vi "Plate Tank 3.vi"() -> ()   [LabVIEW 2019]
uses:
  <vilib>/NI/Current Value Table/Type Defs/Single Tag.ctl
  <vilib>/NI/Current Value Table/Type Defs/Data Types.ctl
  <vilib>/Utility/sysdir.llb/System Directory Type.ctl
  <vilib>/NI/STM/TCP/Read Meta Data (TCP Ref).vi
  <vilib>/NI/STM/TCP/Get Connection Reference (TCP).vi
  <vilib>/NI/AMC/Read Termination Message.vi
  <vilib>/NI/AMC/Create Single Message.vi
  <vilib>/NI/AMC/Update Message Routing Info.vi
  <vilib>/NI/STM/TCP/Read Meta Data (TCP Clst).vi
  <vilib>/NI/AMC/Send Message.vi
  <vilib>/NI/AMC/Globals.vi
  <userlib>/_OpenG.lib/comparison/comparison.llb/I32 Changed__ogtk.vi
  <vilib>/NI/STM/TCP/Write Message (TCP).vi
  <vilib>/NI/AMC/AMC.lvlib
  <vilib>/NI/STM/NI STM.lvlib
  <vilib>/NI/Current Value Table/Current Value Table.lvlib
panel:
  in  "EZ Recipe Button":bool
  out "Loaded Recipe":string
  in  "Load A Recipe":bool
  in  "Save This Recipe":bool
  out "Right Time":dbl format="%.1f"
  out "Left Time":dbl format="%.1f"
  out "Total Amp*min R":dbl format="%.1f"
  out "Total Amp*min L":dbl format="%.1f"
  in  "Rectifer Settings":i32(listbox)
  in  "MO":string
  in  "BasT1_P Last Hr":bool
  in  "BasT1_Level Last Hr":bool
  out "Boolean 5":bool
  out "SumpBottom":bool
  out "Process 1 Supply":bool
  out "Sump Return":bool
  out "Boolean 2":bool
  out "SG":dbl format="%.3g"
  out "Return to sump 4":bool
  in  "Rectifer Data":enum32{"Standard", "Eng"}(tab)
  out "Current Step":i32
  out "Left Anode Actual Current":dbl(knob) scale=0.0..150.0
  out "Right Anode Actual Current":dbl(knob) scale=0.0..150.0
  out "Left Anode Amp-min":dbl(slide) scale=0.0..800.0
  out "Right Anode Amp-min":dbl(slide) scale=0.0..233.60000610351562
  out "Output Voltage":cluster{dbl, dbl}(graph)
  in  "Tab Control 2":enum32{"Standard", "ENG"}(tab)
  out "Supply Flow":dbl(knob) scale=0.0..65.0
  out "Plating Cell Liquid Level":dbl(slide) scale=0.0..75.0
  out "Cell Temperature":dbl(slide) scale=0.0..60.0
  in  "Cell T Last Hr":bool
  out "Suck Pump":bool
  out "Suck Pump Flow":dbl format="%#_4g"
  out "SuckPipe":bool
  out "SuckPipe 3":bool
  out "Drain Tee Top":bool
  out "Return to sump 2":bool
  out "Return to sump 3":bool
  out "Flow Controller":dbl(knob) scale=0.0..100.0
  in  "Tab Control":enum32{"Main Pump", "Suck Pump"}(tab)
  out "Amps":dbl format="%#.2g"
  out "Volts":dbl format="%#.1f"
  out "VFD T":dbl format="%#.2g"
  out "RPM":dbl format="%#.0f"
  out "Fault Code":dbl format="%#.2g"
  out "Freq":dbl format="%#.2g"
  out "SP1 Amps":dbl caption="Amps" format="%#.2g"
  out "SP1 Volts":dbl caption="Volts" format="%#.1g"
  out "SP1 RPM":dbl caption="RPM" format="%#.2g"
  out "SP1 VFD T":dbl caption="VFD T" format="%#.2g"
  out "SP1 Fault Code":dbl caption="Fault Code" format="%#.2g"
  out "SP1 Freq":dbl caption="Freq" format="%#.2g"
  out "Flow 1":dbl format="%#_4g"
  out "Flow 2":dbl format="%#_4g"
  out "Flow 3":dbl format="%#_4g"
  out "Flow 4":dbl format="%#_4g"
  out "Return to sump":bool
  out "E Stop":bool
  out "Run Enabled?":bool
  in  "Full Drain Plating Cell":bool
  out "Rack Motion":bool
  out "Right Eductor Motion":bool
  out "Left Eductor Motion":bool
  out "Right Output On":bool
  in  "Enable Rack Motion":bool
  in  "Rack RPM":dbl(knob) scale=0.0..15.0
  out "Left Output On":bool
  in  "Start Cycle":bool
  in  "Cancel Cycle":bool
  out "SuckPipe 2":bool
  out "Main Pump":bool
  in  "Enable Eductor Motion":bool
  in  "Eductor RPM":dbl(knob) scale=0.0..15.0
  in  "Supply Pressure (kPa)":dbl(knob)=50.0 min=50.0 max=200.0 step=5.0 scale=50.0..200.0
  in  "Total Inflow (L/min)":dbl(knob)=40.0 min=25.0 max=50.0 step=0.5 scale=25.0..50.0
  in  "Suck Pump fraction of inflow":dbl(knob)=5.0 min=5.0 max=90.0 step=1.0 scale=0.0..90.0
  out "Sump Level":dbl(slide) scale=0.0..1000.0
  out "Supply Pressure":dbl(knob) scale=0.0..200.0
  in  "Enable Suck Pump":bool
  in  "Enable Plating Cell":bool
  in  "Machine":bool
  in  "Basement 4":bool
  in  "Dryer":bool
  in  "Rinse 4":bool
  in  "Rinse 3":bool
  in  "Rinse 2":bool
  in  "Basement 3":bool
  in  "Basement 2":bool
  in  "Basement 1":bool
  in  "Plater 6":bool
  in  "Plater 5":bool
  in  "Plater 4":bool
  in  "Plater 3":bool
  in  "Plater 2":bool
  in  "Plater 1":bool
  in  "Predip":bool
  in  "Rinse 1":bool
  in  "Cleaner":bool
  in  "Etch":bool
  out "status":string
  out "Boolean 4":bool
  # "Module Selection"
  # "Rectifier Settings"
  # "Recipe"
  # "Fluid Flow Control"
  # "Rectifier Control"
  # "Rectifier Output"
  # "Motion starts when rectifiers cycle"
  # "Note: RPM settings shared with tank 4"
  # "kPa"
  # "@"
  # "Output"
  # "cm"
  # "°C"
  # "L/min"
  # "cm"
  # "L/min"
  # "L/min"
  # "L/min"
  # "L/min"
  # "L/min"
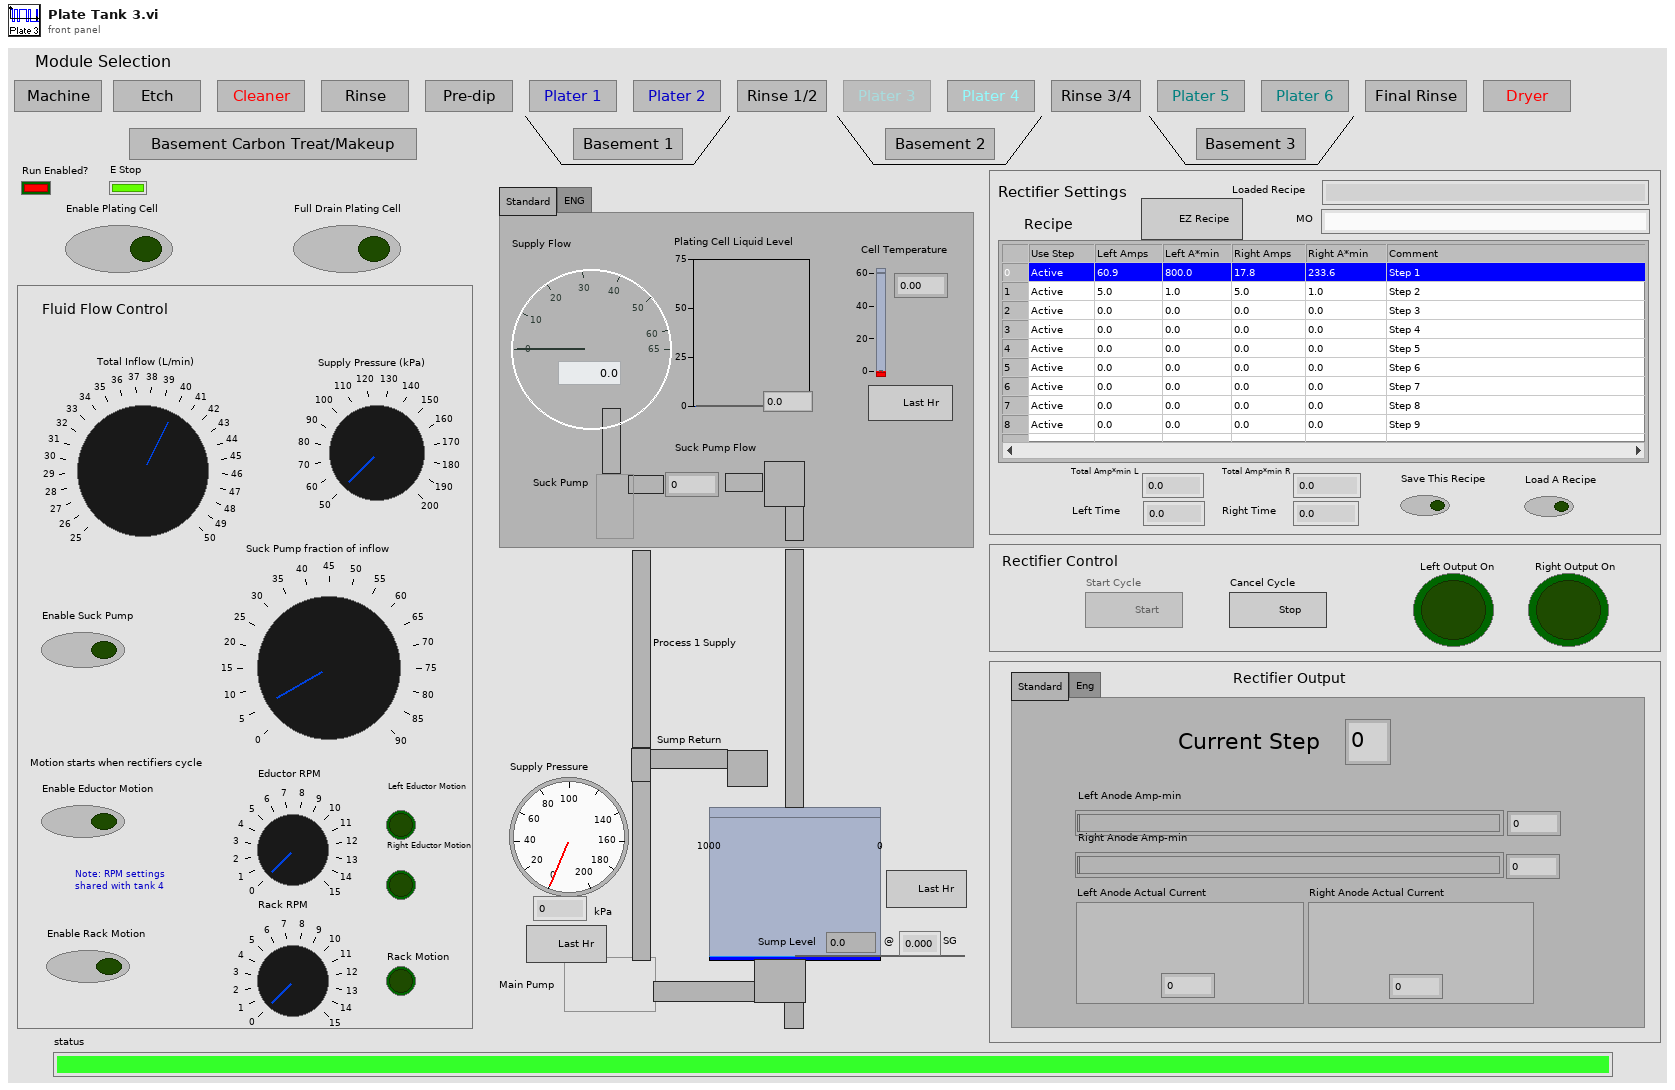
[diagram p1: front panel]
types:
  T1 = typedef "Current Value Table.lvlib/Single Tag.ctl" = cluster{"Data Type":T2, "Name":string, "Value":string, "Description":string}
  T2 = typedef "Current Value Table.lvlib/Data Types.ctl" = enum16{"Double", "Single", "I64", "I32", "I16", "I8", "U64", "U32", "U16", "U8", "String", "Boolean", "Array of U8", "Array of U16", "Array of U32", "Array of U64", "Array of I64", "Array of I32", "Array of I16", "Array of I8", "Array of Double", "Array of Single", "Array of Boolean", "Array of String"}
  T3 = typedef "NI STM.lvlib/TCP Connection Info.ctl" = cluster{"connection ID":refnum<k5>, "meta data":T4[]}
  T4 = typedef "NI STM.lvlib/MetaDataElement.ctl" = string
  T5 = typedef "AMC.lvlib/Message Queue.ctl" = refnum<queue>
  T6 = cluster{"Shift":bool, "Ctrl":bool, "Alt":bool, "Cmd":bool, "Opt":bool}
  T7 = typedef "LVPoint32TypeDef.ctl" = cluster{"Horizontal":i32, "Vertical":i32}
  T8 = typedef "LVRowAndColumnTypeDef.ctl" = cluster{"Row":i32, "Column":i32}
  T9 = enum8{"Enabled", "Disabled", "Disabled and Grayed Out"}
  T10 = typedef "System Directory Type.ctl" = i32
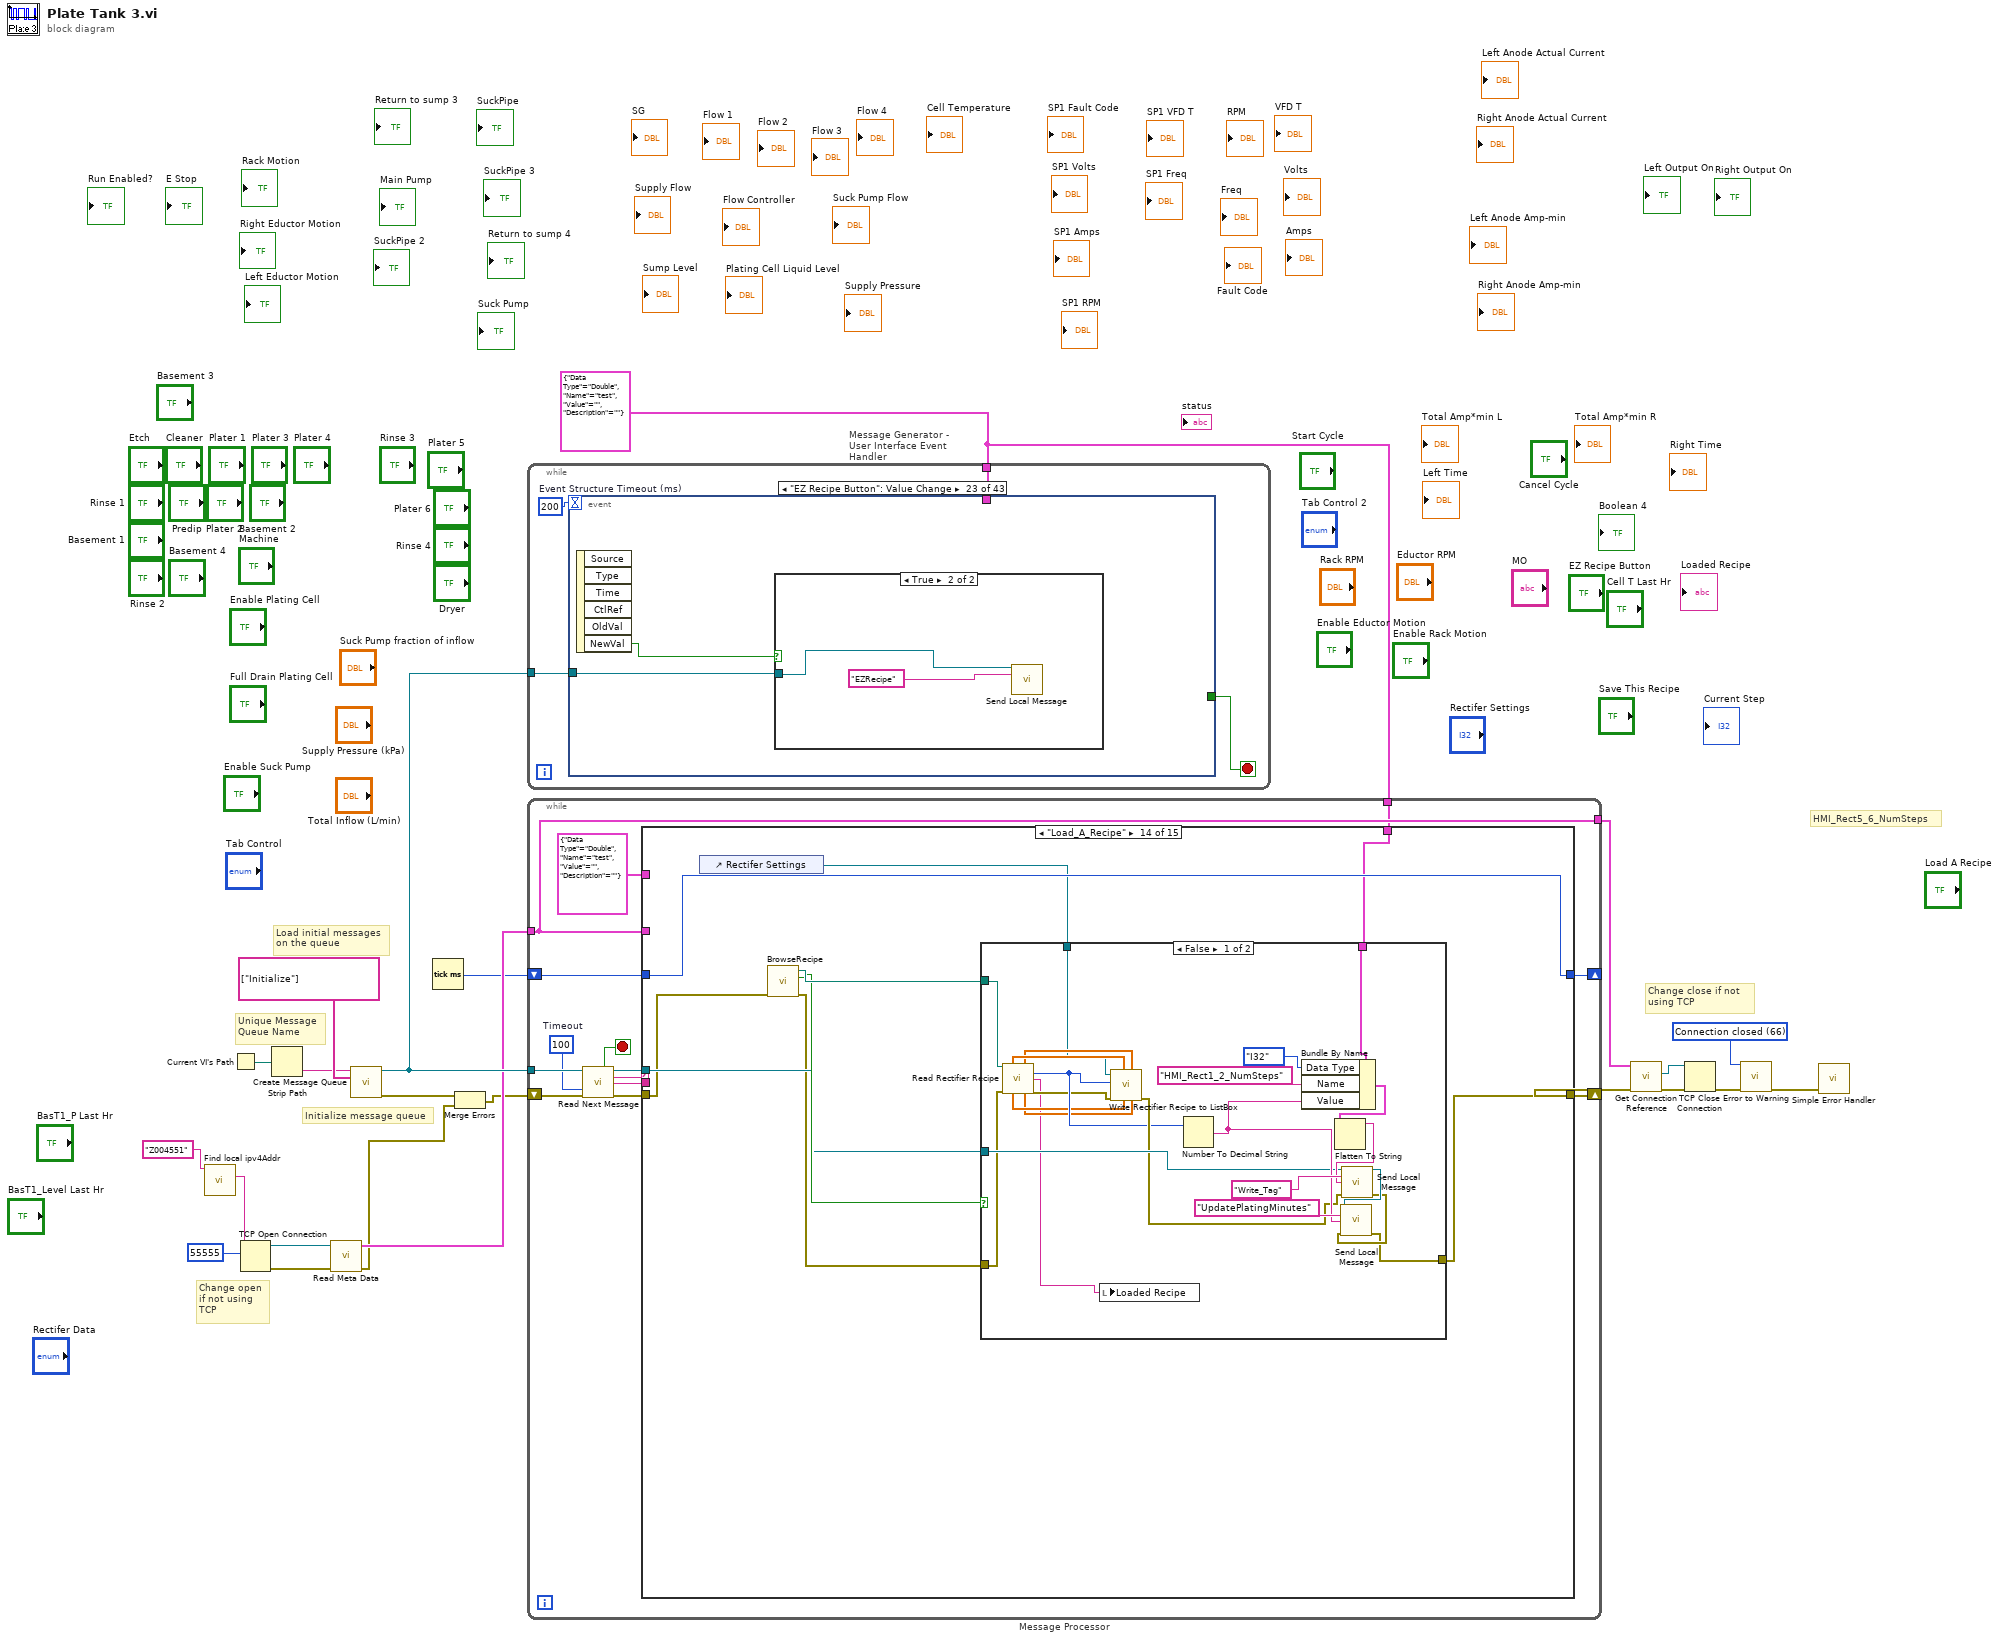
[diagram p0: block diagram]
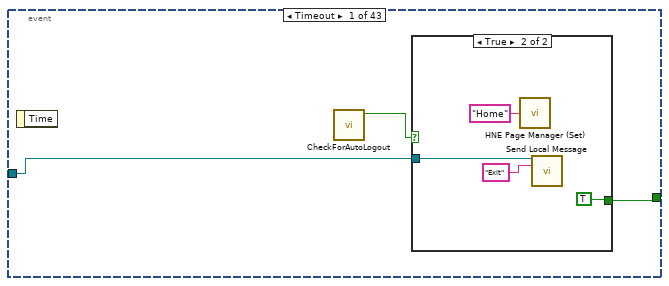
[diagram p2: hidden frame]
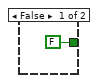
[diagram p3: hidden frame]
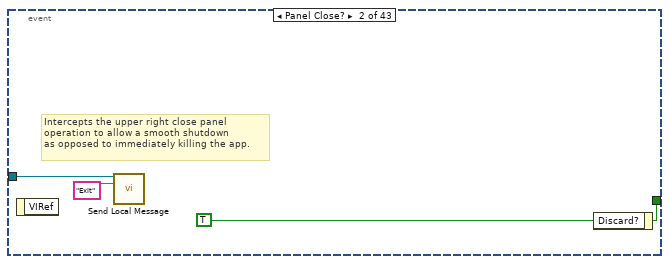
[diagram p4: hidden frame]
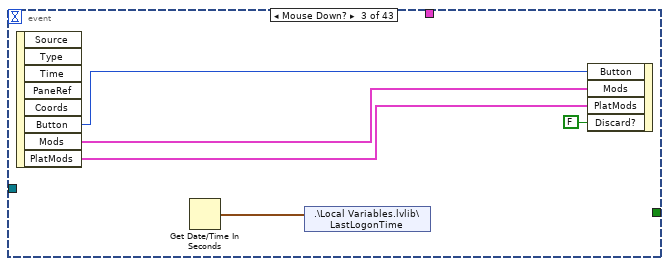
[diagram p5: hidden frame]
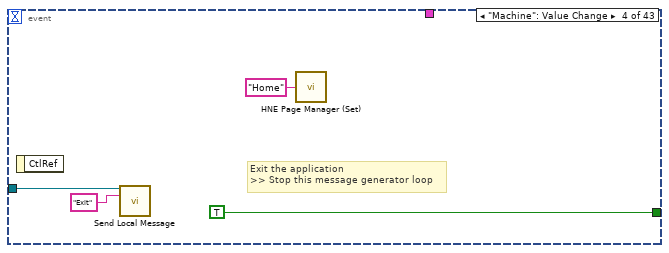
[diagram p6: hidden frame]
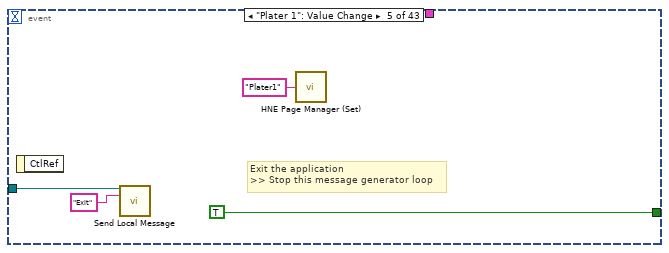
[diagram p7: hidden frame]
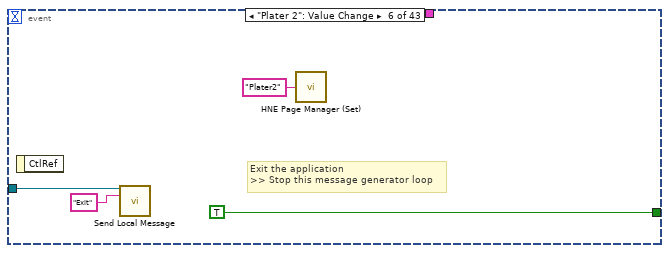
[diagram p8: hidden frame]
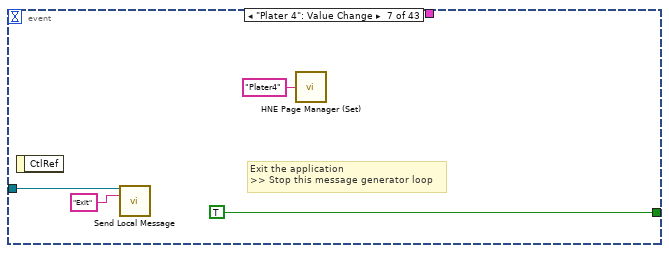
[diagram p9: hidden frame]
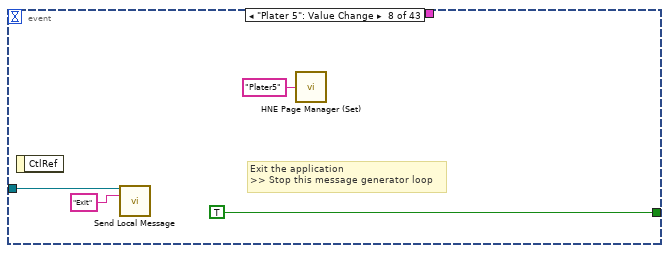
[diagram p10: hidden frame]
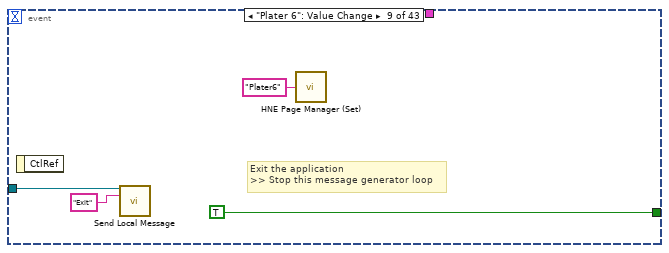
[diagram p11: hidden frame]
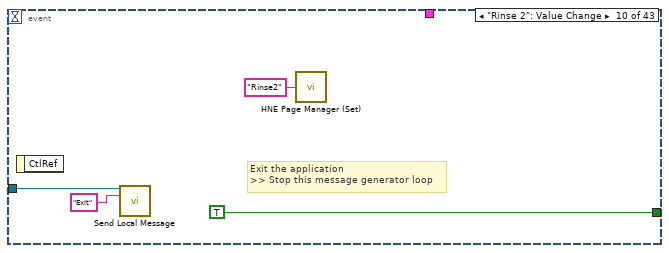
[diagram p12: hidden frame]
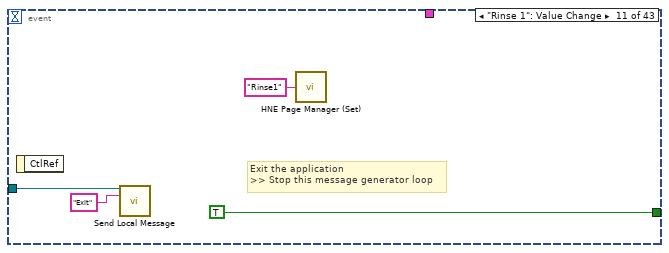
[diagram p13: hidden frame]
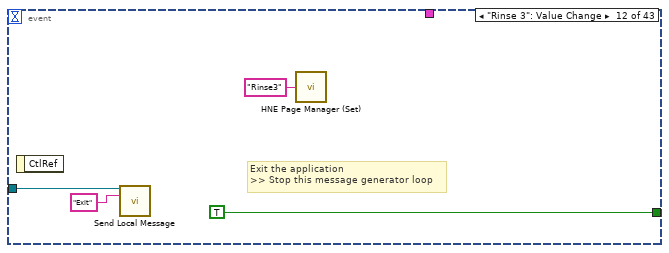
[diagram p14: hidden frame]
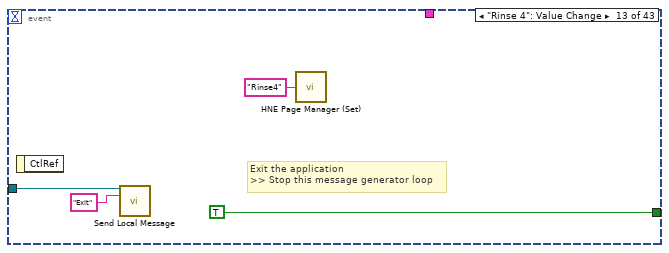
[diagram p15: hidden frame]
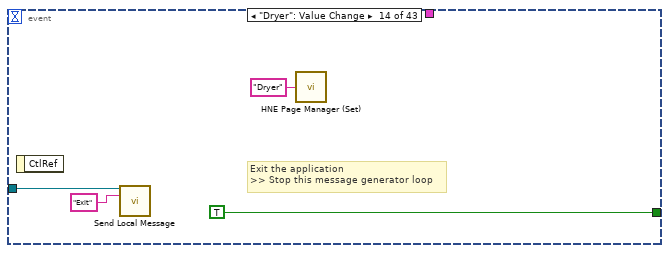
[diagram p16: hidden frame]
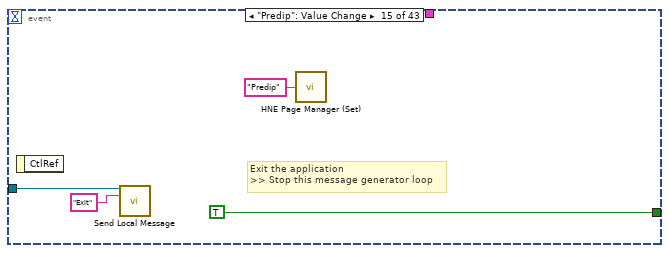
[diagram p17: hidden frame]
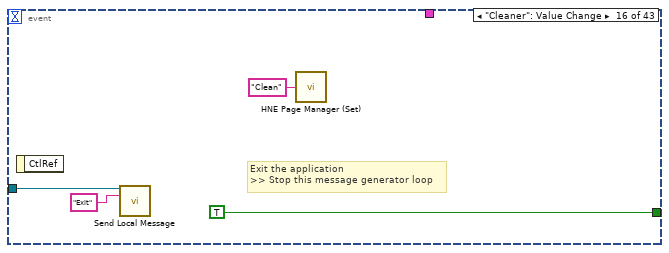
[diagram p18: hidden frame]
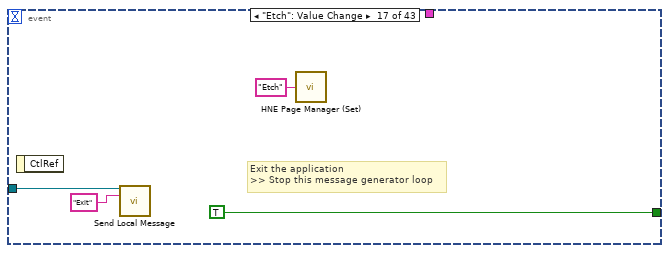
[diagram p19: hidden frame]
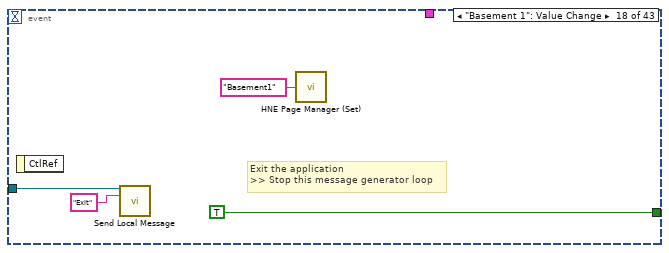
[diagram p20: hidden frame]
diagram:
  w1 = T1 {"Data Type"=enum."Double", "Name"="test", "Value"="", "Description"=""} ("Tag")
  w13 = 66 items=["No Error", "Argument Error", "Memory Full", "Out of Zone", "End of File", "File Already Open", "Generic File IO Error", "File Not Found", "File Permission Error", "Disk Full", "Duplicate Path", "Too Many Files Open", "Not Enabled", "Resource File Not Found", "Cannot Add Resource", "Resource Not Found", "Image Not Found", "Image Memory Error", "Pen Does Not Exist", "Config Bad Type", "Config Token Not Found", "Config Parse Error", "Config Memory Error", "Bad External Code Format", "Bad External Code Offset", "External Code Not Present", "Null Window", "Destroy Window Mixup", "Null Menu", "Print Aborted", "Bad Print Record", "Print Driver Error", "Windows Error During Print", "Memory Error During Print", "Print Dialog Error", "Generic Print Error", "Invalid Device Refnum", "Device Not Found", "Device Parameter Error", "Device Unit Error", "Can't Open Device", "Device Call Aborted", "Generic Error", "Cancelled By User", "Object ID Too Low", "Object ID Too High", "Object Not In Heap", "Unknown Heap", "Bad DefProc ID", "DefProc Not In Table", "Message Out Of Range", "Null Method", "Unknown Message", "Manager Call Not Supported", "Bad address", "Connection In progress", "Connection timed out", "Connection is already in progress", "Network attribute not supported", "Network error", "Address in use", "System out of memory", "Connection aborted", "Connection refused", "Connection is not connected", "Connection is already connected", "Connection closed", "Initialize error (interapplication manager)", "Bad occurrence", "Wait on unbound occurrence handler", "Occurrence queue overflow", "Bad path", "Semaphore not signaled", "Unrecognized type (interapplication manager)"] ("1st Error to Convert")
  # "HMI_Rect5_6_NumSteps"
  # "Change close if not using TCP"
  # "Change open if not using TCP"
  # "Initialize message queue"
  # "Unique Message\nQueue Name"
  # "Load initial messages\non the queue"
  n1 = call "Find local ipv4Addr.vi"("MachineToFind"="Z004551" ("Target IP Address")) -> ("name"=w5:string)  [unwired: 9 in, 1 out]
  n2 = Current VI's Path() -> (path=w19:path)
  n3 = TCP Open Connection(address=w5, remote port or service name=u16 55555 ("remote port")) -> (connection ID=w17:refnum<k5>, error out=w16:errorcluster)  [unwired: 1 in, 2 out]
  n4 = Strip Path(path=w19) -> (name=w21:string)  [unwired: 1 out]
  n5 = call-poly <vilib>:"Read Meta Data.vi"("error in"=w16, "connection ID"=w17) -> ("error out"=w3:errorcluster, "connection info out"=w15:T3)  [unwired: 7 in, 1 out]
  n6 = call <vilib>:"Create Message Queue.vi"("message queue name"=w21, "initial message names"=string[] ["Initialize"]) -> ("message queue out"=w20:T5, "error out"=w4:errorcluster)  [unwired: 12 in]
  n7 = Tick Count (ms)() -> (millisecond timer value=w7:u32)
  n8 = Merge Errors(w4, w3) -> (w2:errorcluster)
  n9 = while "Message Generator - User Interface Event Handler" {
    tunnel: w20 -> [w24]
    tunnel: w1 -> [w23]
    stop <- w25 stop-if-true
    w26 = 200  # Event Structure Timeout (ms)
    n10 = event shown="[22] \"EZ Recipe Button\": Value Change" {
      selector: _ -> [_ _ _ _ _ _ _ _ _ _ _ _ _ _ _ _ _ _ _ _ _ _ _ _ _ _ _ _ _ _ _ _ _ _ _ _ _ _ _ _ _ _ _]
      dyn-events: _ -> [_ _ _ _ _ _ _ _ _ _ _ _ _ _ _ _ _ _ _ _ _ _ _ _ _ _ _ _ _ _ _ _ _ _ _ _ _ _ _ _ _ _ _]
      timeout: w26 -> [_ _ _ _ _ _ _ _ _ _ _ _ _ _ _ _ _ _ _ _ _ _ _ _ _ _ _ _ _ _ _ _ _ _ _ _ _ _ _ _ _ _ _]
      tunnel: [w29 w37 _ TRUE ("Discard?") TRUE ("Discard?") TRUE ("Discard?") TRUE ("Discard?") TRUE ("Discard?") TRUE ("Discard?") TRUE ("Discard?") TRUE ("Discard?") TRUE ("Discard?") TRUE ("Discard?") TRUE ("Discard?") TRUE ("Discard?") TRUE ("Discard?") TRUE ("Discard?") TRUE ("Discard?") TRUE ("Discard?") TRUE ("Discard?") TRUE ("Discard?") FALSE ("Discard?") _ FALSE ("Discard?") FALSE ("Discard?") FALSE ("Discard?") FALSE ("Discard?") FALSE ("Discard?") FALSE ("Discard?") FALSE ("Discard?") FALSE ("Discard?") FALSE ("Discard?") FALSE ("Discard?") FALSE ("Discard?") FALSE ("Discard?") FALSE ("Discard?") _ _ _ _ _ _ _] -> w25
      tunnel: w24 -> [w28 w35 _ w44 w48 w52 w56 w60 w64 w68 w72 w76 w80 w84 w88 w92 w96 w100 w104 w108 w112 w118 w120 w125 w130 w143 w154 w165 w176 w180 w194 w214 w224 w234 w244 w256 w258 w260 w265 w270 w277 w295 _]
      tunnel: w23 -> [_ _ _ _ _ _ _ _ _ _ _ _ _ _ _ _ _ _ _ _ _ _ _ _ _ w140 w151 w162 w173 w179 w193 w213 w223 w233 w243 w255 _ _ _ _ w276 _ _]
      event Timeout {
        n11 = event-data() -> ()  [unwired: 2 out]
        n12 = call "CheckForAutoLogout.vi"() -> ("Boolean"=w27:bool)  [unwired: 11 in]
        n13 = case shown="True" w27 {
          tunnel: [FALSE ("Discard?") TRUE ("Discard?")] -> w29
          tunnel: w28 -> [_ w31]
          frame False {
          }
          frame True {
            n14 = call <userlib>:"HNE Page Manager (Set).vi"("Next Page"="Home") -> ()  [unwired: 4 in, 1 out]
            n15 = call <vilib>:"Send Local Message.vi"("message queue in"=w31, "message name"="Exit") -> ()  [unwired: 11 in, 3 out]
          }
        }
      }
      event Panel Close? {
        w37 = TRUE ("Discard?")
        # "Intercepts the upper right close panel\noperation to allow a smooth shutdown\nas opposed to immediately killing the app."
        n16 = event-data() -> ()  [unwired: 2 out]
        n17 = call <vilib>:"Send Local Message.vi"("message queue in"=w35, "message name"="Exit") -> ()  [unwired: 11 in, 3 out]
        n18 = event-data("Discard?"=w37) -> ()  [unwired: 1 in, 1 out]
      }
      event Mouse Down? {
        n19 = event-data() -> ("Button"=w41:u16, "Mods"=w40:cluster{"Double Click":bool, "Menu Key":bool}, "PlatMods"=w39:T6)  [unwired: 6 out]
        n20 = Get Date/Time In Seconds() -> (seconds since 1Jan1904=w38:timestamp)
        n21 = shared-variable ".\\Local Variables.lvlib\\LastLogonTime"(w38) -> ()  [unwired: 1 in, 1 out]
        n22 = event-data("Button"=w41, "Mods"=w40, "PlatMods"=w39, "Discard?"=FALSE) -> ()  [unwired: 1 in, 1 out]
      }
      event "Machine": Value Change {
        # "Exit the application\n>> Stop this message generator loop"
        n23 = event-data() -> ()  [unwired: 2 out]
        n24 = call <vilib>:"Send Local Message.vi"("message queue in"=w44, "message name"="Exit") -> ()  [unwired: 11 in, 3 out]
        n25 = call <userlib>:"HNE Page Manager (Set).vi"("Next Page"="Home") -> ()  [unwired: 4 in, 1 out]
      }
      event "Plater 1": Value Change {
        # "Exit the application\n>> Stop this message generator loop"
        n26 = event-data() -> ()  [unwired: 2 out]
        n27 = call <vilib>:"Send Local Message.vi"("message queue in"=w48, "message name"="Exit") -> ()  [unwired: 11 in, 3 out]
        n28 = call <userlib>:"HNE Page Manager (Set).vi"("Next Page"="Plater1") -> ()  [unwired: 4 in, 1 out]
      }
      event "Plater 2": Value Change {
        # "Exit the application\n>> Stop this message generator loop"
        n29 = event-data() -> ()  [unwired: 2 out]
        n30 = call <vilib>:"Send Local Message.vi"("message queue in"=w52, "message name"="Exit") -> ()  [unwired: 11 in, 3 out]
        n31 = call <userlib>:"HNE Page Manager (Set).vi"("Next Page"="Plater2") -> ()  [unwired: 4 in, 1 out]
      }
      event "Plater 4": Value Change {
        # "Exit the application\n>> Stop this message generator loop"
        n32 = event-data() -> ()  [unwired: 2 out]
        n33 = call <vilib>:"Send Local Message.vi"("message queue in"=w56, "message name"="Exit") -> ()  [unwired: 11 in, 3 out]
        n34 = call <userlib>:"HNE Page Manager (Set).vi"("Next Page"="Plater4") -> ()  [unwired: 4 in, 1 out]
      }
      event "Plater 5": Value Change {
        # "Exit the application\n>> Stop this message generator loop"
        n35 = event-data() -> ()  [unwired: 2 out]
        n36 = call <vilib>:"Send Local Message.vi"("message queue in"=w60, "message name"="Exit") -> ()  [unwired: 11 in, 3 out]
        n37 = call <userlib>:"HNE Page Manager (Set).vi"("Next Page"="Plater5") -> ()  [unwired: 4 in, 1 out]
      }
      event "Plater 6": Value Change {
        # "Exit the application\n>> Stop this message generator loop"
        n38 = event-data() -> ()  [unwired: 2 out]
        n39 = call <vilib>:"Send Local Message.vi"("message queue in"=w64, "message name"="Exit") -> ()  [unwired: 11 in, 3 out]
        n40 = call <userlib>:"HNE Page Manager (Set).vi"("Next Page"="Plater6") -> ()  [unwired: 4 in, 1 out]
      }
      event "Rinse 2": Value Change {
        # "Exit the application\n>> Stop this message generator loop"
        n41 = event-data() -> ()  [unwired: 2 out]
        n42 = call <vilib>:"Send Local Message.vi"("message queue in"=w68, "message name"="Exit") -> ()  [unwired: 11 in, 3 out]
        n43 = call <userlib>:"HNE Page Manager (Set).vi"("Next Page"="Rinse2") -> ()  [unwired: 4 in, 1 out]
      }
      event "Rinse 1": Value Change {
        # "Exit the application\n>> Stop this message generator loop"
        n44 = event-data() -> ()  [unwired: 2 out]
        n45 = call <vilib>:"Send Local Message.vi"("message queue in"=w72, "message name"="Exit") -> ()  [unwired: 11 in, 3 out]
        n46 = call <userlib>:"HNE Page Manager (Set).vi"("Next Page"="Rinse1") -> ()  [unwired: 4 in, 1 out]
      }
      event "Rinse 3": Value Change {
        # "Exit the application\n>> Stop this message generator loop"
        n47 = event-data() -> ()  [unwired: 2 out]
        n48 = call <vilib>:"Send Local Message.vi"("message queue in"=w76, "message name"="Exit") -> ()  [unwired: 11 in, 3 out]
        n49 = call <userlib>:"HNE Page Manager (Set).vi"("Next Page"="Rinse3") -> ()  [unwired: 4 in, 1 out]
      }
      event "Rinse 4": Value Change {
        # "Exit the application\n>> Stop this message generator loop"
        n50 = event-data() -> ()  [unwired: 2 out]
        n51 = call <vilib>:"Send Local Message.vi"("message queue in"=w80, "message name"="Exit") -> ()  [unwired: 11 in, 3 out]
        n52 = call <userlib>:"HNE Page Manager (Set).vi"("Next Page"="Rinse4") -> ()  [unwired: 4 in, 1 out]
      }
      event "Dryer": Value Change {
        # "Exit the application\n>> Stop this message generator loop"
        n53 = event-data() -> ()  [unwired: 2 out]
        n54 = call <vilib>:"Send Local Message.vi"("message queue in"=w84, "message name"="Exit") -> ()  [unwired: 11 in, 3 out]
        n55 = call <userlib>:"HNE Page Manager (Set).vi"("Next Page"="Dryer") -> ()  [unwired: 4 in, 1 out]
      }
      event "Predip": Value Change {
        # "Exit the application\n>> Stop this message generator loop"
        n56 = event-data() -> ()  [unwired: 2 out]
        n57 = call <vilib>:"Send Local Message.vi"("message queue in"=w88, "message name"="Exit") -> ()  [unwired: 11 in, 3 out]
        n58 = call <userlib>:"HNE Page Manager (Set).vi"("Next Page"="Predip") -> ()  [unwired: 4 in, 1 out]
      }
      event "Cleaner": Value Change {
        # "Exit the application\n>> Stop this message generator loop"
        n59 = event-data() -> ()  [unwired: 2 out]
        n60 = call <vilib>:"Send Local Message.vi"("message queue in"=w92, "message name"="Exit") -> ()  [unwired: 11 in, 3 out]
        n61 = call <userlib>:"HNE Page Manager (Set).vi"("Next Page"="Clean") -> ()  [unwired: 4 in, 1 out]
      }
      event "Etch": Value Change {
        # "Exit the application\n>> Stop this message generator loop"
        n62 = event-data() -> ()  [unwired: 2 out]
        n63 = call <vilib>:"Send Local Message.vi"("message queue in"=w96, "message name"="Exit") -> ()  [unwired: 11 in, 3 out]
        n64 = call <userlib>:"HNE Page Manager (Set).vi"("Next Page"="Etch") -> ()  [unwired: 4 in, 1 out]
      }
      event "Basement 1": Value Change {
        # "Exit the application\n>> Stop this message generator loop"
        n65 = event-data() -> ()  [unwired: 2 out]
        n66 = call <vilib>:"Send Local Message.vi"("message queue in"=w100, "message name"="Exit") -> ()  [unwired: 11 in, 3 out]
        n67 = call <userlib>:"HNE Page Manager (Set).vi"("Next Page"="Basement1") -> ()  [unwired: 4 in, 1 out]
      }
      event "Basement 2": Value Change {
        # "Exit the application\n>> Stop this message generator loop"
        n68 = event-data() -> ()  [unwired: 2 out]
        n69 = call <vilib>:"Send Local Message.vi"("message queue in"=w104, "message name"="Exit") -> ()  [unwired: 11 in, 3 out]
        n70 = call <userlib>:"HNE Page Manager (Set).vi"("Next Page"="Basement2") -> ()  [unwired: 4 in, 1 out]
      }
      event "Basement 3": Value Change {
        # "Exit the application\n>> Stop this message generator loop"
        n71 = event-data() -> ()  [unwired: 2 out]
        n72 = call <vilib>:"Send Local Message.vi"("message queue in"=w108, "message name"="Exit") -> ()  [unwired: 11 in, 3 out]
        n73 = call <userlib>:"HNE Page Manager (Set).vi"("Next Page"="Basement3") -> ()  [unwired: 4 in, 1 out]
      }
      event "Basement 4": Value Change {
        # "Exit the application\n>> Stop this message generator loop"
        n74 = event-data() -> ()  [unwired: 2 out]
        n75 = call <vilib>:"Send Local Message.vi"("message queue in"=w112, "message name"="Exit") -> ()  [unwired: 11 in, 3 out]
        n76 = call <userlib>:"HNE Page Manager (Set).vi"("Next Page"="Basement4") -> ()  [unwired: 4 in, 1 out]
      }
      event "Enable Plating Cell": Value Change {
        n77 = event-data() -> ("NewVal"=w116:bool)  [unwired: 1 out]
        n78 = call "Validate Plate Tank Enable.vi"("Valve No."=139, "Test Value"=w116, "Tag"="HMI_Tank3_Enable", "Queue in"=w118) -> ()  [unwired: 8 in]
      }
      event "EZ Recipe Button": Value Change {
        n79 = event-data() -> ("NewVal"=w121:bool)  [unwired: 6 out]
        n80 = case shown="True" w121 {
          tunnel: w120 -> [_ w122]
          frame False {
          }
          frame True {
            n81 = call <vilib>:"Send Local Message.vi"("message queue in"=w122, "message name"="EZRecipe") -> ()  [unwired: 11 in, 3 out]
          }
        }
      }
      event "Save This Recipe": Value Change {
        n82 = event-data() -> ("NewVal"=w124:bool)  [unwired: 1 out]
        n83 = case shown="True" w124 {
          tunnel: w125 -> [_ w127]
          frame False {
          }
          frame True {
            n84 = call <vilib>:"Send Local Message.vi"("message queue in"=w127, "message name"="Save_Recipe") -> ()  [unwired: 11 in, 3 out]
          }
        }
      }
      event "Load A Recipe": Value Change {
        n85 = event-data() -> ("NewVal"=w129:bool)  [unwired: 1 out]
        n86 = case shown="True" w129 {
          tunnel: w130 -> [_ w132]
          frame False {
          }
          frame True {
            n87 = call <vilib>:"Send Local Message.vi"("message queue in"=w132, "message name"="Load_A_Recipe") -> ()  [unwired: 11 in, 3 out]
          }
        }
      }
      event "Full Drain Plating Cell": Value Change {
        n88 = event-data() -> ("NewVal"=w142:bool)  [unwired: 1 out]
        n89 = Boolean To (0,1)(Boolean=w142) -> (0, 1=w141:i16)
        n90 = Number To Decimal String(number=w141) -> (decimal integer string=w137:string)  [unwired: 1 in]
        n91 = Bundle By Name(cluster=w140, "Data Type"=Data_Types."Boolean", "Name"="HMI_Tank3_Drain", "Value"=w137) -> (w136:T1)
        n92 = Flatten To String(anything=w136) -> (data string=w135:string)  [unwired: 3 in, 2 out]
        n93 = call <vilib>:"Send Local Message.vi"("message queue in"=w143, "message name"="Write_Tag", "message value"=w135) -> ()  [unwired: 10 in, 3 out]
      }
      event "Enable Eductor Motion": Value Change {
        n94 = event-data() -> ("NewVal"=w153:bool)  [unwired: 1 out]
        n95 = Boolean To (0,1)(Boolean=w153) -> (0, 1=w152:i16)
        n96 = Number To Decimal String(number=w152) -> (decimal integer string=w148:string)  [unwired: 1 in]
        n97 = Bundle By Name(cluster=w151, "Data Type"=Data_Types."Boolean", "Name"="HMI_Tank3_Eductor_Motors_Run", "Value"=w148) -> (w147:T1)
        n98 = Flatten To String(anything=w147) -> (data string=w146:string)  [unwired: 3 in, 2 out]
        n99 = call <vilib>:"Send Local Message.vi"("message queue in"=w154, "message name"="Write_Tag", "message value"=w146) -> ()  [unwired: 10 in, 3 out]
      }
      event "Enable Rack Motion": Value Change {
        n100 = event-data() -> ("NewVal"=w164:bool)  [unwired: 1 out]
        n101 = Boolean To (0,1)(Boolean=w164) -> (0, 1=w163:i16)
        n102 = Number To Decimal String(number=w163) -> (decimal integer string=w159:string)  [unwired: 1 in]
        n103 = Bundle By Name(cluster=w162, "Data Type"=Data_Types."Boolean", "Name"="HMI_Tank3_Rack_Motor_Run", "Value"=w159) -> (w158:T1)
        n104 = Flatten To String(anything=w158) -> (data string=w157:string)  [unwired: 3 in, 2 out]
        n105 = call <vilib>:"Send Local Message.vi"("message queue in"=w165, "message name"="Write_Tag", "message value"=w157) -> ()  [unwired: 10 in, 3 out]
      }
      event "Enable Suck Pump": Value Change {
        n106 = event-data() -> ("NewVal"=w175:bool)  [unwired: 1 out]
        n107 = Boolean To (0,1)(Boolean=w175) -> (0, 1=w174:i16)
        n108 = Number To Decimal String(number=w174) -> (decimal integer string=w170:string)  [unwired: 1 in]
        n109 = Bundle By Name(cluster=w173, "Data Type"=Data_Types."Boolean", "Name"="HMI_Tnk3_Enable_SuckPump", "Value"=w170) -> (w169:T1)
        n110 = Flatten To String(anything=w169) -> (data string=w168:string)  [unwired: 3 in, 2 out]
        n111 = call <vilib>:"Send Local Message.vi"("message queue in"=w176, "message name"="Write_Tag", "message value"=w168) -> ()  [unwired: 10 in, 3 out]
      }
      event "Start Cycle": Value Change {
        n112 = event-data() -> ("NewVal"=w178:bool)  [unwired: 1 out]
        n113 = case shown="True" w178 {
          tunnel: w180 -> [_ w191]
          tunnel: w178 -> [_ w190]
          tunnel: w179 -> [_ w188]
          frame False {
          }
          frame True {
            n114 = Boolean To (0,1)(Boolean=w190) -> (0, 1=w189:i16)
            n115 = Number To Decimal String(number=w189) -> (decimal integer string=w185:string)  [unwired: 1 in]
            n116 = Bundle By Name(cluster=w188, "Data Type"=Data_Types."Boolean", "Name"="HMI_Rect5_6_Cycle", "Value"=w185) -> (w184:T1)
            n117 = Flatten To String(anything=w184) -> (data string=w183:string)  [unwired: 3 in, 2 out]
            n118 = call <vilib>:"Send Local Message.vi"("message queue in"=w191, "message name"="Write_Tag", "message value"=w183) -> ()  [unwired: 10 in, 3 out]
          }
        }
      }
      event "Cancel Cycle": Value Change {
        n119 = event-data() -> ("NewVal"=w192:bool)  [unwired: 1 out]
        n120 = case shown="True" w192 {
          tunnel: w194 -> [_ w205]
          tunnel: w192 -> [_ w204]
          tunnel: w193 -> [_ w202]
          frame False {
          }
          frame True {
            n121 = Boolean To (0,1)(Boolean=w204) -> (0, 1=w203:i16)
            n122 = Number To Decimal String(number=w203) -> (decimal integer string=w199:string)  [unwired: 1 in]
            n123 = Bundle By Name(cluster=w202, "Data Type"=Data_Types."Boolean", "Name"="HMI_Rect5_6_CycleStop", "Value"=w199) -> (w198:T1)
            n124 = Flatten To String(anything=w198) -> (data string=w197:string)  [unwired: 3 in, 2 out]
            n125 = call <vilib>:"Send Local Message.vi"("message queue in"=w205, "message name"="Write_Tag", "message value"=w197) -> ()  [unwired: 10 in, 3 out]
          }
        }
      }
      event "Eductor RPM": Value Change {
        n126 = event-data() -> ("NewVal"=w207:dbl)  [unwired: 1 out]
        n127 = Number To Fractional String(number=w207) -> (F-format string=w206:string)  [unwired: 3 in]
        n128 = Bundle By Name(cluster=w213, "Data Type"=Data_Types."Double", "Name"="HMI_Tnk3_Eductor_RPM", "Value"=w206) -> (w210:T1)
        n129 = Flatten To String(anything=w210) -> (data string=w209:string)  [unwired: 3 in, 2 out]
        n130 = call <vilib>:"Send Local Message.vi"("message queue in"=w214, "message name"="Write_Tag", "message value"=w209) -> ()  [unwired: 10 in, 3 out]
      }
      event "Rack RPM": Value Change {
        n131 = event-data() -> ("NewVal"=w217:dbl)  [unwired: 1 out]
        n132 = Number To Fractional String(number=w217) -> (F-format string=w216:string)  [unwired: 3 in]
        n133 = Bundle By Name(cluster=w223, "Data Type"=Data_Types."Double", "Name"="HMI_Tnk3_Rack_RPM", "Value"=w216) -> (w220:T1)
        n134 = Flatten To String(anything=w220) -> (data string=w219:string)  [unwired: 3 in, 2 out]
        n135 = call <vilib>:"Send Local Message.vi"("message queue in"=w224, "message name"="Write_Tag", "message value"=w219) -> ()  [unwired: 10 in, 3 out]
      }
      event "Total Inflow (L/min)": Value Change {
        n136 = event-data() -> ("NewVal"=w227:dbl)  [unwired: 1 out]
        n137 = Number To Fractional String(number=w227) -> (F-format string=w226:string)  [unwired: 3 in]
        n138 = Bundle By Name(cluster=w233, "Data Type"=Data_Types."Double", "Name"="HMI_TNK3_Flow_Setpoint", "Value"=w226) -> (w230:T1)
        n139 = Flatten To String(anything=w230) -> (data string=w229:string)  [unwired: 3 in, 2 out]
        n140 = call <vilib>:"Send Local Message.vi"("message queue in"=w234, "message name"="Write_Tag", "message value"=w229) -> ()  [unwired: 10 in, 3 out]
      }
      event "Supply Pressure (kPa)": Value Change {
        n141 = event-data() -> ("NewVal"=w237:dbl)  [unwired: 1 out]
        n142 = Number To Fractional String(number=w237) -> (F-format string=w236:string)  [unwired: 3 in]
        n143 = Bundle By Name(cluster=w243, "Data Type"=Data_Types."Double", "Name"="HMI_BAS_TNK2_P_Setpoint", "Value"=w236) -> (w240:T1)
        n144 = Flatten To String(anything=w240) -> (data string=w239:string)  [unwired: 3 in, 2 out]
        n145 = call <vilib>:"Send Local Message.vi"("message queue in"=w244, "message name"="Write_Tag", "message value"=w239) -> ()  [unwired: 10 in, 3 out]
      }
      event "Suck Pump fraction of inflow": Value Change {
        n146 = event-data() -> ("NewVal"=w247:dbl)  [unwired: 1 out]
        n147 = Divide(x=w247, y=100.0) -> (x/y=w246:dbl)
        n148 = Number To Fractional String(number=w246) -> (F-format string=w249:string)  [unwired: 3 in]
        n149 = Bundle By Name(cluster=w255, "Data Type"=Data_Types."Double", "Name"="HMI_TNK3_SuckPmpFrac_Setpoint", "Value"=w249) -> (w252:T1)
        n150 = Flatten To String(anything=w252) -> (data string=w251:string)  [unwired: 3 in, 2 out]
        n151 = call <vilib>:"Send Local Message.vi"("message queue in"=w256, "message name"="Write_Tag", "message value"=w251) -> ()  [unwired: 10 in, 3 out]
      }
      event Menu Selection (User) {
        # "Add run-time menu items to the message\nqueue. The message handler case names must match the menu ItemTag names."
        n152 = event-data() -> ("ItemTag"=w259:string)  [unwired: 1 out]
        n153 = call <vilib>:"Send Local Message.vi"("message queue in"=w258, "message name"=w259) -> ()  [unwired: 11 in, 3 out]
      }
      event "Cell T Last Hr": Value Change {
        n154 = event-data() -> ("NewVal"=w261:bool)  [unwired: 3 out]
        n155 = case shown="True" w261 {
          tunnel: w260 -> [_ w264]
          frame False {
          }
          frame True {
            n156 = call <vilib>:"Send Local Message.vi"("message queue in"=w264, "message name"="DisplayLastHr", "message value"="TNK3_Temperature") -> ()  [unwired: 10 in, 3 out]
          }
        }
      }
      event "BasT1_Level Last Hr": Value Change {
        n157 = event-data() -> ("NewVal"=w266:bool)  [unwired: 3 out]
        n158 = case shown="True" w266 {
          tunnel: w265 -> [_ w269]
          frame False {
          }
          frame True {
            n159 = call <vilib>:"Send Local Message.vi"("message queue in"=w269, "message name"="DisplayLastHr", "message value"="BAS_Proc2_Tank_Level") -> ()  [unwired: 10 in, 3 out]
          }
        }
      }
      event "BasT1_P Last Hr": Value Change {
        n160 = event-data() -> ("NewVal"=w271:bool)  [unwired: 3 out]
        n161 = case shown="True" w271 {
          tunnel: w270 -> [_ w274]
          frame False {
          }
          frame True {
            n162 = call <vilib>:"Send Local Message.vi"("message queue in"=w274, "message name"="DisplayLastHr", "message value"="TNK34_MainPressure") -> ()  [unwired: 10 in, 3 out]
          }
        }
      }
      event "Rectifer Settings": Mouse Down {
        n163 = event-data() -> ("CtlRef"=w281:refnum<vi>, "Coords"=w279:T7, "Button"=w280:u16)  [unwired: 6 out]
        n164 = call "Handle Rectifer Step Selection.vi"("Coords"=w279, "Button"=w280, "MulticolumnListbox in"=w281) -> ("Row"=w275:i32)  [unwired: 8 in]
        n165 = Greater Than 0?(x=w275) -> (x > 0?=w278:bool)
        n166 = case shown="True" w278 {
          tunnel: w277 -> [_ w284]
          tunnel: w276 -> [_ w283]
          tunnel: w275 -> [_ w282]
          frame False {
          }
          frame True {
            n167 = Number To Decimal String(number=w282) -> (decimal integer string=w285:string)  [unwired: 1 in]
            n168 = Bundle By Name(cluster=w283, "Data Type"=Data_Types."I32", "Name"="HMI_Rect5_6_NumSteps", "Value"=w285) -> (w289:T1)
            n169 = Flatten To String(anything=w289) -> (data string=w288:string)  [unwired: 3 in, 2 out]
            n170 = call <vilib>:"Send Local Message.vi"("message queue in"=w284, "message name"="Write_Tag", "message value"=w288) -> ("message queue out"=w287:T5)  [unwired: 10 in, 2 out]
            n171 = call <vilib>:"Send Local Message.vi"("message queue in"=w287, "message name"="UpdatePlatingMinutes", "message value"=w285) -> ()  [unwired: 10 in, 3 out]
          }
        }
      }
      event "Rectifer Settings": Edit Cell {
        n172 = event-data() -> ("CtlRef"=w299:refnum<vi>, "String"=w298:string, "Coords"=w297:T8)  [unwired: 4 out]
        n173 = call "Data Check DC Rectifier Settings.vi"("String"=w298, "Coords"=w297, "MulticolumnListbox in"=w299) -> ("error out"=w294:errorcluster)  [unwired: 7 in, 1 out]
        n174 = shared-variable-read(refnum<k21> "ni.var.psp://z004551/CDL0100 ReadWriteTags/HMI_Rect5_6_NumSteps" ("shared variable refnum in"), 0) -> (w300:i32)  [unwired: 1 in, 3 out]
        n175 = Number To Decimal String(number=w300) -> (decimal integer string=w293:string)  [unwired: 1 in]
        n176 = call <vilib>:"Send Local Message.vi"("message queue in"=w295, "message name"="UpdatePlatingMinutes", "message value"=w293, "error in"=w294) -> ()  [unwired: 9 in, 3 out]
      }
      event "MO": Value Change {
        n177 = event-data() -> ("NewVal"=w303:string)  [unwired: 6 out]
        n178 = shared-variable ".\\Local Variables.lvlib\\PT3_MO"(w303) -> ()  [unwired: 1 in, 1 out]
      }
    }
  }
  n179 = while "Message Processor" {
    shift-left: w2 -> [w313]
    shift-right: [w317] -> w8
    tunnel: w20 -> [w314]
    tunnel: w15 -> [w308]
    tunnel: [w308] -> w9
    shift-right: [w305] -> _
    shift-left: w7 -> [w306]
    tunnel: w1 -> [w304]
    stop <- w316 stop-if-true
    w309 = 100  # Timeout
    n180 = call <vilib>:"Read Next Message.vi"("message queue in"=w314, "timeout (1 ms)"=w309, "error in"=w313) -> ("exit process?"=w316:bool, "message queue out"=w315:T5, "message name"=w311:string, "message value"=w310:string, "error out"=w312:errorcluster)  [unwired: 5 in, 3 out]
    n181 = case shown="\"Load_A_Recipe\"" w311 {
      selector: w311 -> [_ _ w409 _ _ _ _ _ _ _ _ _ _ _ _]
      tunnel: w315 -> [_ _ _ _ _ _ w525 _ _ _ _ w546 _ w572 w602]
      tunnel: w312 -> [w318 w330 w410 w411 w413 w415 w526 w528 w532 w535 w537 w550 w564 w568 w601]
      tunnel: [w318 w330 w410 errorcluster {"status"=FALSE, "code"=0, "source"=""} ("error out") w413 w415 w524 w528 w531 w535 w537 w549 w555 w567 w600] -> w317
      tunnel: w310 -> [_ _ _ _ _ _ _ _ w530 _ w539 w541 _ _ _]
      tunnel: w308 -> [_ _ _ _ _ _ _ _ w533 _ _ _ _ _ _]
      tunnel: T1 {"Data Type"=enum."Double", "Name"="test", "Value"="", "Description"=""} ("Tag") -> [_ _ _ _ _ _ _ _ _ _ _ _ _ _ _]
      tunnel: w306 -> [_ w325 _ _ _ w414 _ _ w529 w536 w538 _ w554 w575 _]
      tunnel: [_ w326 _ _ _ w414 _ _ w529 w536 w538 _ w554 w575 _] -> w305
      tunnel: w304 -> [_ _ _ _ _ _ _ _ _ _ _ _ _ w569 w612]
      frame "---------- Framework Operations ----------" {
        # "Dummy case to add a seperator in the Case Structure menu"
      }
      frame "", "Idle" {
        n182 = stacked-sequence {
          frame #0 {
            n183 = control-ref of="Enable Plating Cell"() -> (w336:refnum<vi>)
            n184 = shared-variable-read(refnum<k21> "ni.var.psp://z004551/CDL0100 ReadTags/Tnk3_Can_Plate" ("shared variable refnum in"), FALSE) -> (w346:bool)  [unwired: 1 in, 3 out]
            n185 = shared-variable-read(refnum<k21> "ni.var.psp://z004551/CDL0100 ReadWriteTags/HMI_Tank4_Enable" ("shared variable refnum in"), FALSE) -> (w333:bool)  [unwired: 1 in, 3 out]
            n186 = shared-variable-read(refnum<k21> "ni.var.psp://z004551/CDL0100 ReadWriteTags/HMI_Enable_BTnk2_Pump" ("shared variable refnum in"), FALSE) -> (w338:bool)  [unwired: 1 in, 3 out]
            n187 = shared-variable-read(refnum<k21> "ni.var.psp://z004551/CDL0100 ReadWriteTags/HMI_Tank3_Enable" ("shared variable refnum in"), FALSE) -> (w332:bool)  [unwired: 1 in, 3 out]
            n188 = Or(x=w333, y=w332) -> (x .or. y?=w331:bool)
            n189 = Or(x=w331, y=w338) -> (x .or. y?=w341:bool)
            n190 = case shown="False" w346 {
              tunnel: [T9."Disabled and Grayed Out" ("Disabled") T9."Enabled" ("Disabled")] -> w347
              frame False {
              }
              frame True {
              }
            }
            n191 = call "GrayOutButtonFromPSPVar.vi"("shared variable refnum in"=refnum<k21> "ni.var.psp://z004551/CDL0100 ReadWriteTags/HMI_Tank3_Drain", "Boolean in"=w336) -> ()  [unwired: 10 in]
            n192 = case shown="True" w341 {
              tunnel: [T9."Enabled" ("Disabled") T9."Disabled and Grayed Out" ("Disabled")] -> w340
              frame False {
              }
              frame True {
              }
            }
            n193 = control-ref of="Full Drain Plating Cell"() -> (w339:refnum<vi>)
            n194 = control-ref of="Start Cycle"() -> (w348:refnum<vi>)
            n195 = property class="Bool (strict)"(reference=w348, "DisabledEnum"=w347) -> ()  [unwired: 1 in, 2 out]
            n196 = property class="Bool (strict)"(reference=w339, "DisabledEnum"=w340) -> ()  [unwired: 1 in, 2 out]
          }
          frame #1 {
            n197 = shared-variable-read(refnum<k21> "ni.var.psp://z004551/CDL0100 ReadTags/IO_Bas_Tnk2_3Way_At_Recirc" ("shared variable refnum in"), FALSE) -> (w358:bool)  [unwired: 1 in, 3 out]
            n198 = shared-variable-read(refnum<k21> "ni.var.psp://z004551/CDL0100 ReadTags/IO_Bas_Tnk2_3Way_At_Open" ("shared variable refnum in"), FALSE) -> (w359:bool)  [unwired: 1 in, 3 out]
            n199 = shared-variable-read(refnum<k21> "ni.var.psp://z004551/CDL0100 ReadTags/IO_Bas_Tnk2_3Way_At_Closed" ("shared variable refnum in"), FALSE) -> (w362:bool)  [unwired: 1 in, 3 out]
            n200 = Or(x=w359, y=w358) -> (x .or. y?=w356:bool)
            "Sump Return" <- w356
            "Boolean 2" <- w356
            n201 = Or(x=w362, y=w359) -> (x .or. y?=w357:bool)
            "Return to sump" <- w357
            "Drain Tee Top" <- w357
            "Return to sump 2" <- w357
            "Process 1 Supply" <- w357
            n202 = Or(x=w357, y=w356) -> (x .or. y?=→"Boolean 5":bool)
          }
          frame #2 {
            n203 = shared-variable-read(refnum<k21> "ni.var.psp://z004551/CDL0100 ReadWriteTags/HMI_Tank3_Drain" ("shared variable refnum in"), FALSE) -> (w367:bool)  [unwired: 1 in, 3 out]
            n204 = shared-variable-read(refnum<k21> "ni.var.psp://z004551/CDL0100 ReadWriteTags/HMI_Enable_BTnk2_Pump" ("shared variable refnum in"), FALSE) -> (w368:bool)  [unwired: 1 in, 3 out]
            n205 = Or(x=w368, y=w367) -> (x .or. y?=→"SumpBottom":bool)
          }
          frame #3 {
            n206 = shared-variable-read(refnum<k21> "ni.var.psp://z004551/CDL0100 ReadTags/Rect5_6_CurrRecpStp" ("shared variable refnum in"), 0) -> (w374:i32)  [unwired: 1 in, 3 out]
            n207 = call-poly <userlib>:"Data Changed__ogtk.vi"("I32"=w374) -> ("Changed"=w375:bool)
            n208 = case shown="True" w375 {
              tunnel: w374 -> [_ w379]
              frame False {
              }
              frame True {
                w384 = 0.0 ("Scale.Range:Minimum")
                n209 = shared-variable-read(refnum<k21> "ni.var.psp://z004551/CDL0100 ReadWriteTags/HMI_Rect5_6_NumSteps" ("shared variable refnum in"), 0) -> (w378:i32)  [unwired: 1 in, 3 out]
                n210 = Less?(x=w379, y=w378) -> (x < y?=w391:bool)
                n211 = case shown="False" w391 {
                  tunnel: w379 -> [w396 w397]
                  tunnel: [w395 w397] -> w385
                  frame False {
                    n212 = Decrement(x=w396) -> (x-1=w395:i32)
                  }
                  frame True {
                  }
                }
                n213 = shared-variable-read(refnum<k21> "ni.var.psp://z004551/CDL0100 ReadWriteTags/HMI_Rct6_AMin_SetPnts" ("shared variable refnum in"), dbl[] []) -> (w386:dbl[])  [unwired: 1 in, 3 out]
                n214 = Index Array(array=w386, index=w385) -> (element=w382:dbl)
                n215 = shared-variable-read(refnum<k21> "ni.var.psp://z004551/CDL0100 ReadWriteTags/HMI_Rct5_AMin_SetPnts" ("shared variable refnum in"), dbl[] []) -> (w389:dbl[])  [unwired: 1 in, 3 out]
                n216 = Index Array(array=w389, index=w385) -> (element=w383:dbl)
                n217 = control-ref of="Right Anode Amp-min"() -> (w381:refnum<vi>)
                n218 = control-ref of="Left Anode Amp-min"() -> (w380:refnum<vi>)
                n219 = property class="Slide (strict)"(reference=w380, "Scale.Maximum"=w383, "Scale.Minimum"=w384) -> ()  [unwired: 1 in, 2 out]
                n220 = property class="Slide (strict)"(reference=w381, "Scale.Maximum"=w382, "Scale.Minimum"=w384) -> ()  [unwired: 1 in, 2 out]
              }
            }
          }
        }
        n221 = local read "Left Output On"() -> (w322:bool)
        n222 = local read "Right Output On"() -> (w323:bool)
        n223 = control-ref of="status"() -> (w329:refnum<vi>)
        n224 = Tick Count (ms)() -> (millisecond timer value=w324:u32)
        n225 = Subtract(x=w324, y=w325) -> (x-y=w327:u32)
        n226 = call <userlib>:"TAE Format Alarm Ticker.vi"("Alarm Ticker Ref"=w329) -> ()  [unwired: 15 in]
        n227 = Or(x=w322, y=w323) -> (x .or. y?=w321:bool)
        n228 = Greater?(x=w327, y=u32 500) -> (0:w320:bool)
        n229 = And(x=w321, y=w320) -> (x .and. y?=w319:bool)
        n230 = case shown="True" w319 {
          tunnel: w324 -> [_ w399]
          tunnel: [w398 w399] -> w326
          tunnel: w325 -> [w398 _]
          frame False {
          }
          frame True {
            n231 = shared-variable-read(refnum<k21> "ni.var.psp://z004551/CDL0100 ReadTags/Rect5_ActlVolts" ("shared variable refnum in"), 0.0) -> (w402:dbl)  [unwired: 1 in, 3 out]
            n232 = shared-variable-read(refnum<k21> "ni.var.psp://z004551/CDL0100 ReadTags/Rect6_ActlVolts" ("shared variable refnum in"), 0.0) -> (w401:dbl)  [unwired: 1 in, 3 out]
            n233 = Bundle(w402, w401) -> (→"Output Voltage":cluster{dbl, dbl})  [unwired: 1 in]
          }
        }
      }
      frame "Missing Message Handler", Default {
        # "Call this case if a message is received that is not handled \nby any other case. Typically this is a programming error\nas a result of a typo or unhandled message/missing message handler."
        n234 = Format Into String(format string="DevError: Missing message handler for '%s\" message." ("message"), w409) -> (resulting string=w407:string)  [unwired: 2 in, 1 out]
        n235 = One Button Dialog(message=w407) -> ()  [unwired: 2 out]
      }
      frame "Error" {
        # "General Error Case - this case is called if an error is passed using the error cluster below. Typically most new errors should be handed in each individual case and not passed in the rror cluster. If necessary a custom error handler case should be added and called from other cases."
        n236 = call <vilib>:"Simple Error Handler.vi"("error in (no error)"=w411) -> ()  [unwired: 1 in, 8 out]
      }
      frame "---------- Generic Operations ----------" {
        # "Dummy case to add a seperator in the Case Structure menu"
      }
      frame "Initialize" {
        n237 = stacked-sequence {
          seq-local: [_ w433 _ _ _] -> [_ _ w451 w477 w503]
          seq-local: [_ _ w449 _ _] -> [_ _ _ w469 w511]
          seq-local: [_ _ w448 _ _] -> [_ _ _ w474 w506]
          frame #0 {
            n238 = shared-variable-read(refnum<k21> "ni.var.psp://z004551/CDL0100 ReadWriteTags/HMI_TNK3_SuckPmpFrac_Setpoint" ("shared variable refnum in"), 0.0) -> (w418:dbl)  [unwired: 1 in, 3 out]
            n239 = shared-variable-read(refnum<k21> "ni.var.psp://z004551/CDL0100 ReadWriteTags/HMI_Tnk3_Enable_SuckPump" ("shared variable refnum in"), FALSE) -> (w421:bool)  [unwired: 1 in, 3 out]
            n240 = shared-variable-read(refnum<k21> "ni.var.psp://z004551/CDL0100 ReadWriteTags/HMI_Tnk3_Rack_RPM" ("shared variable refnum in"), 0.0) -> (w432:dbl)  [unwired: 1 in, 3 out]
            n241 = shared-variable-read(refnum<k21> "ni.var.psp://z004551/CDL0100 ReadWriteTags/HMI_Tank3_Rack_Motor_Run" ("shared variable refnum in"), FALSE) -> (w431:bool)  [unwired: 1 in, 3 out]
            n242 = shared-variable-read(refnum<k21> "ni.var.psp://z004551/CDL0100 ReadWriteTags/HMI_TNK3_Flow_Setpoint" ("shared variable refnum in"), 0.0) -> (w430:dbl)  [unwired: 1 in, 3 out]
            n243 = Multiply(x=w418, y=100.0) -> (x*y=w416:dbl)
            n244 = local write "Enable Suck Pump"(w421) -> ()
            n245 = local write "Rack RPM"(w432) -> ()
            n246 = local write "Enable Rack Motion"(w431) -> ()
            n247 = local write "Total Inflow (L/min)"(w430) -> ()
            n248 = local write "Suck Pump fraction of inflow"(w416) -> ()
          }
          frame #1 {
            n249 = shared-variable-read(refnum<k21> "ni.var.psp://z004551/CDL0100 ReadWriteTags/HMI_Tank3_Drain" ("shared variable refnum in"), FALSE) -> (w436:bool)  [unwired: 1 in, 3 out]
            n250 = shared-variable-read(refnum<k21> "ni.var.psp://z004551/CDL0100 ReadWriteTags/HMI_Tnk3_Eductor_RPM" ("shared variable refnum in"), 0.0) -> (w444:dbl)  [unwired: 1 in, 3 out]
            n251 = shared-variable-read(refnum<k21> "ni.var.psp://z004551/CDL0100 ReadWriteTags/HMI_Tank3_Enable" ("shared variable refnum in"), FALSE) -> (w443:bool)  [unwired: 1 in, 3 out]
            n252 = local write "Full Drain Plating Cell"(w436) -> ()
            n253 = shared-variable-read(refnum<k21> "ni.var.psp://z004551/CDL0100 ReadWriteTags/HMI_Tank3_Eductor_Motors_Run" ("shared variable refnum in"), FALSE) -> (w447:bool)  [unwired: 1 in, 3 out]
            n254 = shared-variable-read(refnum<k21> "ni.var.psp://z004551/CDL0100 ReadWriteTags/HMI_Rect5_6_NumSteps" ("shared variable refnum in"), 0) -> (w433:i32)  [unwired: 1 in, 3 out]
            n255 = local write "Enable Plating Cell"(w443) -> ()
            n256 = local write "Eductor RPM"(w444) -> ()
            n257 = local write "Enable Eductor Motion"(w447) -> ()
          }
          frame #2 {
            w452 = 0.0
            n258 = shared-variable ".\\Local Variables.lvlib\\PT3_MO"() -> (w458:string)  [unwired: 1 in, 1 out]
            n259 = shared-variable-read(refnum<k21> "ni.var.psp://z004551/CDL0100 ReadWriteTags/HMI_Rct5_AMin_SetPnts" ("shared variable refnum in"), dbl[] []) -> (w449:dbl[])  [unwired: 1 in, 3 out]
            n260 = shared-variable-read(refnum<k21> "ni.var.psp://z004551/CDL0100 ReadWriteTags/HMI_Rct6_AMin_SetPnts" ("shared variable refnum in"), dbl[] []) -> (w448:dbl[])  [unwired: 1 in, 3 out]
            n261 = shared-variable-read(refnum<k21> "ni.var.psp://z004551/CDL0100 ReadWriteTags/HMI_BAS_TNK2_P_Setpoint" ("shared variable refnum in"), 0.0) -> (w459:dbl)  [unwired: 1 in, 3 out]
            n262 = for {
              N: w451 -> [_]
              tunnel: w448 -> [w464] mode=indexing
              shift-right: [w462] -> w450
              shift-left: w452 -> [w463]
              n263 = Add(x=w464, y=w463) -> (x+y=w462:dbl)
            }
            n264 = for {
              N: w451 -> [_]
              tunnel: w449 -> [w467] mode=indexing
              shift-right: [w465] -> w455
              shift-left: w452 -> [w466]
              n265 = Add(x=w467, y=w466) -> (x+y=w465:dbl)
            }
            n266 = local write "Supply Pressure (kPa)"(w459) -> ()
            n267 = local write "MO"(w458) -> ()
            n268 = local write "Total Amp*min L"(w455) -> ()
            n269 = local write "Total Amp*min R"(w450) -> ()
          }
          frame #3 {
            n270 = Subtract(x=10, y=w477) -> (x-y=w480:i32)
            n271 = Initialize Array(38, w477) -> (w479:i32[])
            n272 = Initialize Array(37, w480) -> (w478:i32[])
            n273 = Build Array (concatenate)(w479, w478) -> (w472:i32[])
            n274 = shared-variable-read(refnum<k21> "ni.var.psp://z004551/CDL0100 ReadWriteTags/HMI_Rct5_A_SetPnts" ("shared variable refnum in"), dbl[] []) -> (w475:dbl[])  [unwired: 1 in, 3 out]
            n275 = shared-variable-read(refnum<k21> "ni.var.psp://z004551/CDL0100 ReadWriteTags/HMI_Rct6_A_SetPnts" ("shared variable refnum in"), dbl[] []) -> (w468:dbl[])  [unwired: 1 in, 3 out]
            n276 = for {
              N: 10 -> [_]
              tunnel: [w502] -> w471 mode=indexing
              tunnel: w475 -> [w499] mode=indexing
              tunnel: w469 -> [w496] mode=indexing
              tunnel: w468 -> [w493] mode=indexing
              tunnel: w474 -> [w491] mode=indexing
              tunnel: [w488] -> w470 mode=indexing
              i -> [w494]
              w490 = i16 1 ("precision (6)")
              n277 = Number To Fractional String(number=w491, precision (6)=w490) -> (F-format string=w489:string)  [unwired: 2 in]
              n278 = Number To Fractional String(number=w493, precision (6)=w490) -> (F-format string=w492:string)  [unwired: 2 in]
              n279 = Number To Fractional String(number=w496, precision (6)=w490) -> (F-format string=w495:string)  [unwired: 2 in]
              n280 = Number To Decimal String(number=w494) -> (decimal integer string=w502:string)  [unwired: 1 in]
              n281 = Number To Fractional String(number=w499, precision (6)=w490) -> (F-format string=w497:string)  [unwired: 2 in]
              n282 = Increment(x=w494) -> (x+1=w500:i32)
              n283 = call "Build Text"("d"=w500) -> ("Result"=w498:string)  [unwired: 13 in, 1 out]
              n284 = Build Array("Active", w497, w495, w492, w489, w498) -> (w488:string[])
            }
            n285 = control-ref of="Rectifer Settings"() -> (w473:refnum<vi>)
            n286 = property class="MCListbox (strict)"(reference=w473, "ItemSyms"=w472, "RowHdrs[]"=w471, "ItemNames"=w470) -> ()  [unwired: 1 in, 2 out]
          }
          frame #4 {
            n287 = control-ref of="Rectifer Settings"() -> (w520:refnum<vi>)
            n288 = control-ref of="Right Anode Amp-min"() -> (w512:refnum<vi>)
            n289 = control-ref of="Left Anode Amp-min"() -> (w513:refnum<vi>)
            n290 = property class="MCListbox (strict)"(reference=w520) -> ("ItemNames"=w519:string[][])  [unwired: 1 in, 2 out]
            n291 = shared-variable-read(refnum<k21> "ni.var.psp://z004551/CDL0100 ReadTags/Rect5_6_CurrRecpStp" ("shared variable refnum in"), 0) -> (w504:i32)  [unwired: 1 in, 3 out]
            n292 = call "Calculate Plating Time DC.vi"("ItemNames"=w519, "Num Steps"=w503) -> ("Right Anode Time"=w517:dbl, "Left Anode Time"=w518:dbl)  [unwired: 8 in]
            n293 = Less?(x=w504, y=w503) -> (x < y?=w514:bool)
            n294 = case shown="False" w514 {
              tunnel: w504 -> [w522 w523]
              tunnel: [w521 w523] -> w507
              frame False {
                n295 = Decrement(x=w522) -> (x-1=w521:i32)
              }
              frame True {
              }
            }
            n296 = local write "Right Time"(w517) -> ()
            n297 = local write "Left Time"(w518) -> ()
            n298 = Index Array(array=w511, index=w507) -> (element=w510:dbl)
            n299 = Index Array(array=w506, index=w507) -> (element=w505:dbl)
            n300 = property class="Slide (strict)"(reference=w513, "Scale.Maximum"=w510, "Scale.Minimum"=0.0 ("Scale.Range:Minimum")) -> ()  [unwired: 1 in, 2 out]
            n301 = property class="Slide (strict)"(reference=w512, "Scale.Maximum"=w505, "Scale.Minimum"=0.0 ("Scale.Range:Minimum")) -> ()  [unwired: 1 in, 2 out]
          }
        }
      }
      frame "Exit" {
        # "Destroy message queue >> this will halt the UI event handler loop"
        # "Stop the VI\n>> Perform any cleanup tasks in this message case.\n>> Clear display before closing."
        n302 = call <vilib>:"Destroy Message Queue.vi"("message queue in"=w525, "error in"=w526) -> ("error out"=w524:errorcluster)  [unwired: 11 in, 2 out]
        n303 = local write "status"("" ("Status")) -> ()
      }
      frame "---------- Application Operations ----------" {
        # "Dummy case to add a seperator in the Case Structure menu"
      }
      frame "Write_Tag" {
        n304 = call-poly <vilib>:"Write Message.vi"("error in"=w532, "data"=w530, "name"="WriteTag", "connection info in"=w533) -> ("error out"=w531:errorcluster)  [unwired: 6 in, 1 out]
      }
      frame "UpdateVPlotX" {
      }
      frame "DisplayLastHr" {
        n305 = call "Trace Variable 1 hour Popup.vi"("Tag"=w539) -> ()  [unwired: 11 in]
      }
      frame "UpdatePlatingMinutes" {
        n306 = Decimal String To Number(string=w541) -> (number=w540:i32)  [unwired: 2 in, 1 out]
        n307 = control-ref of="Rectifer Settings"() -> (w547:refnum<vi>)
        n308 = call "Assemble DC Rectifier Setting Changes for PLC.vi"("Num Steps"=w540, "Rect Number"=5, "error In"=w550, "message queue in"=w546, "MulticolumnListbox in"=w547) -> ("Right Anode Mins"=w542:dbl, "Left Anode Mins"=w543:dbl, "Right AmpMin"=w544:dbl, "Left AmpMin"=w545:dbl, "error out"=w549:errorcluster)  [unwired: 2 in]
        n309 = local write "Total Amp*min L"(w545) -> ()
        n310 = local write "Total Amp*min R"(w544) -> ()
        n311 = local write "Left Time"(w543) -> ()
        n312 = local write "Right Time"(w542) -> ()
      }
      frame "Save_Recipe" {
        n313 = control-ref of="Rectifer Settings"() -> (w565:refnum<vi>)
        n314 = call "Convert DC RectifierListData to Arrays.vi"("error in (no error)"=w564, "MulticolumnListbox in"=w565) -> ("error out"=w556:errorcluster, "Right Amps"=w560:dbl[], "Left Amps"=w561:dbl[], "Right Amp Min"=w557:dbl[], "Left AmpMins"=w558:dbl[])  [unwired: 5 in]
        n315 = shared-variable-read(refnum<k21> "ni.var.psp://z004551/CDL0100 ReadWriteTags/HMI_Rect5_6_NumSteps" ("shared variable refnum in"), 0) -> (w559:i32)  [unwired: 1 in, 3 out]
        n316 = call "Save Rectifier Recipe.vi"("Rev Mult"=0.0, "Right AmpMins"=w557, "Left AmpMins"=w558, "error in"=w556, "Number Steps"=w559, "Right Amps"=w560, "Left Amps"=w561) -> ("error out"=w555:errorcluster, "name"=w551:string, "cancelled"=w552:bool)  [unwired: 2 in]
        n317 = case shown="False" w552 {
          tunnel: w551 -> [w566 _]
          frame False {
            n318 = local write "Loaded Recipe"(w566) -> ()
          }
          frame True {
          }
        }
      }
      frame "Load_A_Recipe" {
        n319 = control-ref of="Rectifer Settings"() -> (w570:refnum<vi>)
        n320 = call "BrowseRecipe.vi"("error in (no error)"=w568) -> ("error out"=w571:errorcluster, "cancelled"=w573:bool, "selected path"=w574:path)  [unwired: 8 in]
        n321 = case shown="False" w573 {
          tunnel: w571 -> [w580 w599]
          tunnel: [w577 w599] -> w567
          tunnel: w572 -> [w590 _]
          tunnel: w569 -> [w589 _]
          tunnel: w574 -> [w579 _]
          tunnel: w570 -> [w578 _]
          frame False {
            n322 = call "Read Rectifier Recipe.vi"("selected path"=w579, "error in"=w580) -> ("Left Amps"=w586:dbl[], "Left AmpMins"=w585:dbl[], "Num Steps"=w584:i32, "name"=w576:string, "Right Amps"=w583:dbl[], "Right AmpMins"=w582:dbl[], "error out"=w581:errorcluster)  [unwired: 5 in, 2 out]
            n323 = local write "Loaded Recipe"(w576) -> ()
            n324 = call "Write Rectifier Recipe to ListBox.vi"("Right AmpMins"=w582, "Left AmpMins"=w585, "Right Amps"=w583, "Left Amps"=w586, "error in (no error)"=w581, "Number Steps"=w584, "ListBox"=w578) -> ("error out"=w588:errorcluster)  [unwired: 4 in]
            n325 = Number To Decimal String(number=w584) -> (decimal integer string=w591:string)  [unwired: 1 in]
            n326 = Bundle By Name(cluster=w589, "Data Type"=Data_Types."I32", "Name"="HMI_Rect1_2_NumSteps", "Value"=w591) -> (w595:T1)
            n327 = Flatten To String(anything=w595) -> (data string=w594:string)  [unwired: 3 in, 2 out]
            n328 = call <vilib>:"Send Local Message.vi"("message queue in"=w590, "message name"="Write_Tag", "message value"=w594, "error in"=w588) -> ("message queue out"=w593:T5, "error out"=w587:errorcluster)  [unwired: 9 in, 1 out]
            n329 = call <vilib>:"Send Local Message.vi"("message queue in"=w593, "message name"="UpdatePlatingMinutes", "message value"=w591, "error in"=w587) -> ("error out"=w577:errorcluster)  [unwired: 9 in, 2 out]
          }
          frame True {
          }
        }
      }
      frame "EZRecipe" {
        w610 = T10 7 items=["User Home"=0, "User Desktop"=1, "User Documents"=2, "User Application Data"=3, "User Preferences"=4, "User Temporary"=5, "Public Documents"=6, "Public Application Data"=7, "Public Preferences"=8, "Public Cache"=13, "System Core Libraries"=9, "System Installed Libraries"=10, "Application Files"=11, "Boot Volume Root"=12] ("system directory type")
        n330 = local read "Loaded Recipe"() -> (w605:string)
        n331 = call <vilib>:"Get System Directory.vi"("system directory type"=w610) -> ("system directory"=w607:path)  [unwired: 10 in]
        n332 = Build Path(base path=w607, name or relative path="TDK\\CDL0100") -> (appended path=w608:path)
        n333 = Build Path(base path=w608, name or relative path=w605) -> (appended path=w606:path)
        n334 = control-ref of="Rectifer Settings"() -> (w611:refnum<vi>)
        n335 = call "CDL0100 Recipe Creator v1.1.vi"("Previous Recipe Path"=w606) -> ("New Recipe Path"=w604:path, "canceled?"=w603:bool)  [unwired: 1 out]
        n336 = case shown="False" w603 {
          tunnel: w601 -> [w617 w636]
          tunnel: [w614 w636] -> w600
          tunnel: w602 -> [w627 _]
          tunnel: w612 -> [w626 _]
          tunnel: w604 -> [w616 _]
          tunnel: w611 -> [w615 _]
          frame False {
            n337 = call "Read Rectifier Recipe.vi"("selected path"=w616, "error in"=w617) -> ("Left Amps"=w623:dbl[], "Left AmpMins"=w622:dbl[], "Num Steps"=w621:i32, "name"=w613:string, "Right Amps"=w620:dbl[], "Right AmpMins"=w619:dbl[], "error out"=w618:errorcluster)  [unwired: 5 in, 2 out]
            n338 = call "Write Rectifier Recipe to ListBox.vi"("Right AmpMins"=w619, "Left AmpMins"=w622, "Right Amps"=w620, "Left Amps"=w623, "error in (no error)"=w618, "Number Steps"=w621, "ListBox"=w615) -> ("error out"=w625:errorcluster)  [unwired: 4 in]
            n339 = local write "Loaded Recipe"(w613) -> ()
            n340 = Number To Decimal String(number=w621) -> (decimal integer string=w628:string)  [unwired: 1 in]
            n341 = Bundle By Name(cluster=w626, "Data Type"=Data_Types."I32", "Name"="HMI_Rect5_6_NumSteps", "Value"=w628) -> (w632:T1)
            n342 = Flatten To String(anything=w632) -> (data string=w631:string)  [unwired: 3 in, 2 out]
            n343 = call <vilib>:"Send Local Message.vi"("message queue in"=w627, "message name"="Write_Tag", "message value"=w631, "error in"=w625) -> ("message queue out"=w630:T5, "error out"=w624:errorcluster)  [unwired: 9 in, 1 out]
            n344 = call <vilib>:"Send Local Message.vi"("message queue in"=w630, "message name"="UpdatePlatingMinutes", "message value"=w628, "error in"=w624) -> ("error out"=w614:errorcluster)  [unwired: 9 in, 2 out]
          }
          frame True {
          }
        }
      }
    }
  }
  n345 = call-poly <vilib>:"Get Connection Reference.vi"("error in"=w8, "connection info in"=w9) -> ("error out"=w12:errorcluster, "connection ID out"=w11:refnum<k5>)  [unwired: 8 out]
  n346 = TCP Close Connection(connection ID=w11, error in (no error)=w12) -> (error out=w14:errorcluster)  [unwired: 2 out]
  n347 = call <vilib>:"Error to Warning.vi"("1st Error to Convert"=w13, "error in"=w14) -> ("warning out"=w10:errorcluster)  [unwired: 3 in, 10 out]
  n348 = call <vilib>:"Simple Error Handler.vi"("error in (no error)"=w10) -> ()  [unwired: 4 in, 5 out]
